vi "Arduino Move To Next Notch.vi"(5 "Ignore Alarm":bool, 7 "Distance":i32, 8 "error in":errorcluster, 9 "Homing Parameters":T1={"Direction (F: CW)"=FALSE, "Speed"=400, "Accel"=400, "Min Distance"=2700, "Short Leg"=0, "Error Cnts"=0}, 10 "Motor":i32, 11 "Addr":refnum<visa-resource-name>) -> (0 "error out":errorcluster, 2 "Actual distance":i32, 3 "Log":string)   [LabVIEW 2024, in "FW Arduino Control.lvclass"]
uses:
  FW Arduino Control.lvclass
  Filter Wheel Arduino Homing cluster.ctl
  da37c6a6-a1a6-4c15-8ebf-7ada4fc6adfa.vi
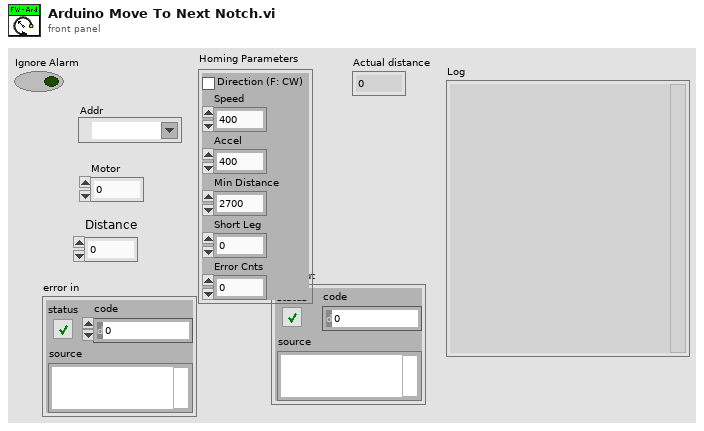
[diagram p1: front panel]
types:
  T1 = typedef "Filter Wheel Arduino Homing cluster.ctl" = cluster{"Direction (F: CW)":bool, "Speed":i32, "Accel":i32, "Min Distance":i32, "Short Leg":i32, "Error Cnts":i32}
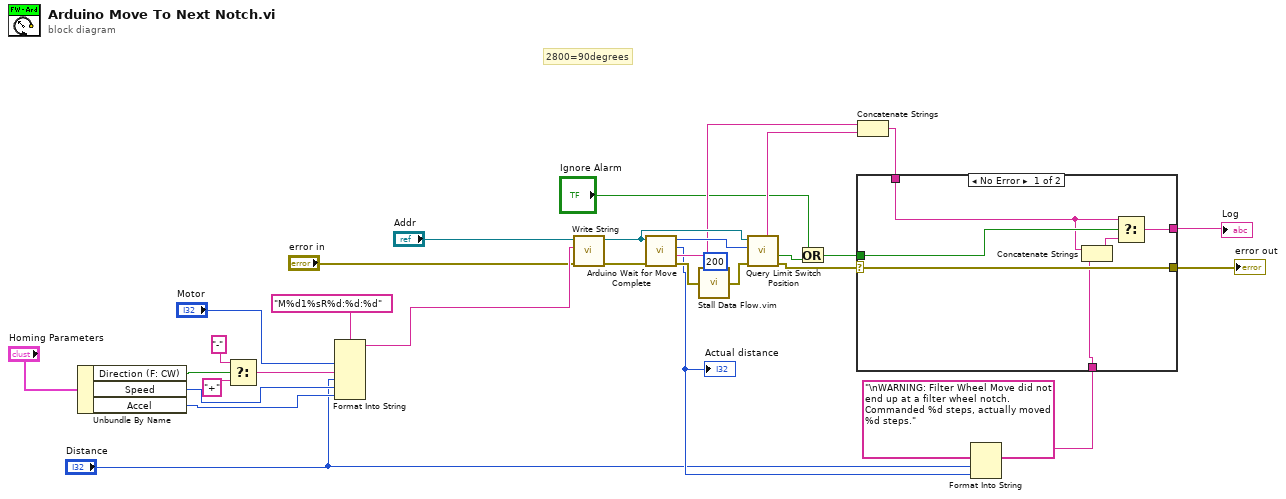
[diagram p0: block diagram]
diagram:
  # "2800=90degrees"
  n1 = Unbundle By Name("Homing Parameters") -> ("Direction (F: CW)"=w22:bool, "Speed"=w19:i32, "Accel"=w21:i32)
  n2 = Select(t="-", s=w22, f="+") -> (s? t:f=w26:string)
  n3 = Format Into String(format string="M%d1%sR%d:%d:%d", "Motor", w26, "Distance", w19, w21) -> (resulting string=w25:string)  [unwired: 2 in, 1 out]
  n4 = call "Write String.vi"("error in (no error)"="error in", "String"=w25, "VISA resource name"="Addr") -> ("error out"=w20:errorcluster, "VISA resource name out"=w17:refnum<visa-resource-name>)  [unwired: 7 in]
  n5 = call "Arduino Wait for Move Complete.vi"("error in (no error)"=w20, "reference"=w17) -> ("error out"=w18:errorcluster, "response"=w14:string, "distance"=w10:i32, "Motor"=w16:i32)  [unwired: 6 in]
  "Actual distance" <- w10
  n6 = call "Stall Data Flow.vim"("value in"=w18, "milliseconds to wait"=u32 200) -> ("value out"=w6:errorcluster)  [unwired: 1 out]
  n7 = call "Query Limit Switch Position.vi"("error in (no error)"=w6, "motor (0:n-1)"=w16, "VISA resource name"=w17) -> ("error out"=w12:errorcluster, "At Switch?"=w13:bool, "response"=w15:string)  [unwired: 4 in, 2 out]
  n8 = Or(x="Ignore Alarm", y=w13) -> (x .or. y?=w4:bool)
  n9 = Concatenate Strings(w14, w15) -> (w2:string)
  n10 = Format Into String(format string="\nWARNING: Filter Wheel Move did not end up at a filter wheel notch. Commanded %d steps, actually moved %d steps.", "Distance", w10) -> (resulting string=w8:string)  [unwired: 2 in, 1 out]
  n11 = case shown="No Error" w12 {
    selector: w12 -> [w37 w39]
    tunnel: w4 -> [w36 _]
    tunnel: w8 -> [w34 _]
    tunnel: [w37 w39] -> w7
    tunnel: w2 -> [w33 w38]
    tunnel: [w32 w38] -> w1
    frame No Error {
      n12 = Concatenate Strings(w33, w34) -> (w35:string)
      n13 = Select(t=w33, s=w36, f=w35) -> (s? t:f=w32:string)
    }
    frame Error {
    }
  }
  "error out" <- w7
  "Log" <- w1
